vi "Get Configuration.vi"(8 "error in (no error)":errorcluster, 11 "Core Plugins Configuration in":refnum<class "Plugin Configuration.lvclass">) -> (0 "error out":errorcluster, 2 "configuration":T1={"name"="", "components"=[], "cycle timing"={"priority"=10000, "decimation"=1, "offset"=0}}, 3 "Core Plugins Configuration out":refnum<class "Plugin Configuration.lvclass">)   [LabVIEW 2019, in "DSF Core.lvlib" / "Plugin Configuration.lvclass"]
uses:
  Plugin Configuration.lvclass
  Typedefs/Core Plugin Configuration.ctl
  Typedefs/DSF Timing Info.ctl
  Plugin Configuration.lvclass/Plugin Configuration.ctl
  DSF Core.lvlib
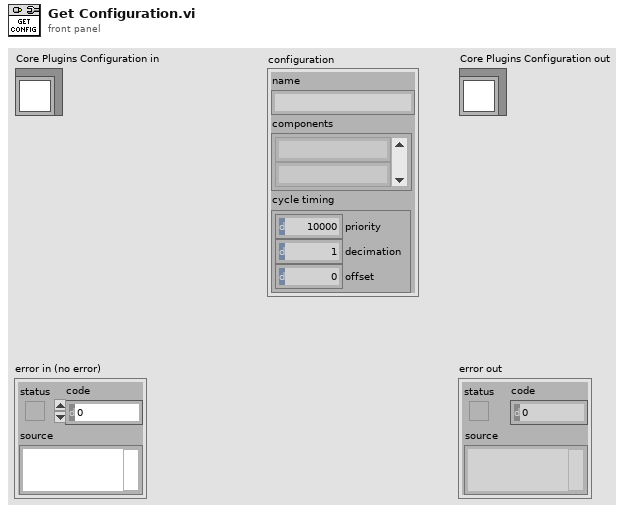
[diagram p1: front panel]
types:
  T1 = typedef "DSF Core.lvlib/Plugin Configuration.lvclass/Core Plugin Configuration.ctl" = cluster{"name":string, "components":string[], "cycle timing":T2}
  T2 = typedef "DSF Core.lvlib/DSF Timing Info.ctl" = cluster{"priority":u64, "decimation":u64, "offset":u64}
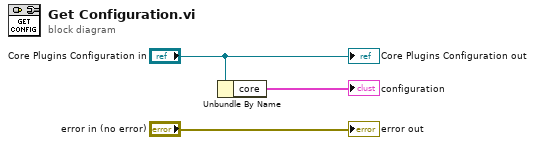
[diagram p0: block diagram]
diagram:
  n1 = Unbundle By Name("Core Plugins Configuration in") -> ("core"=→"configuration":T1)
  "error out" <- "error in (no error)"
  "Core Plugins Configuration out" <- "Core Plugins Configuration in"
